vi "Compute Obstacle Clearance.vi"() -> (0 "obstacle clearance (m)":dbl)   [LabVIEW 2011]
uses:
  Robot Parameters.vi
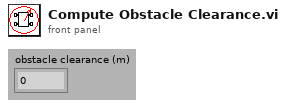
[diagram p1: front panel]
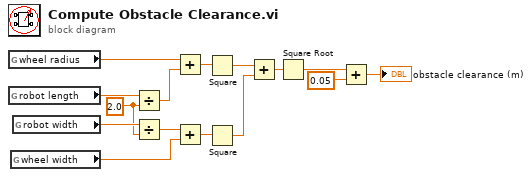
[diagram p0: block diagram]
diagram:
  w1 = 2.0 ("y")
  n1 = global read "Robot Parameters.vi" "wheel radius"() -> (w5:dbl)
  n2 = global read "Robot Parameters.vi" "robot length"() -> (w4:dbl)
  n3 = global read "Robot Parameters.vi" "wheel width"() -> (w2:dbl)
  n4 = global read "Robot Parameters.vi" "robot width"() -> (w3:dbl)
  n5 = Divide(x=w4, y=w1) -> (x/y=w9:dbl)
  n6 = Divide(x=w3, y=w1) -> (x/y=w6:dbl)
  n7 = Add(x=w5, y=w9) -> (x+y=w15:dbl)
  n8 = Add(x=w6, y=w2) -> (x+y=w14:dbl)
  n9 = Square(x=w15) -> (x^2=w11:dbl)
  n10 = Square(x=w14) -> (x^2=w10:dbl)
  n11 = Add(x=w11, y=w10) -> (x+y=w12:dbl)
  n12 = Square Root(x=w12) -> (sqrt(x)=w13:dbl)
  n13 = Add(x=w13, y=0.05) -> (x+y=→"obstacle clearance (m)":dbl)
